vi "GetMeasurements (B fields first).vi"() -> ()   [LabVIEW 2016]
uses:
  <vilib>/Utility/file.llb/Write Delimited Spreadsheet (DBL).vi
panel:
  in  "DVM GIPB Address":string="7"
  out "# of Runs":i32=49
  in  "+B Field Removed?":bool
  out "Remove Field":bool
  out "# of Runs":i32=49
  in  "+B Field Added?":bool
  out "Ready To Change Field":bool
  out "# of Runs":i32
  in  "-B Field Added?":bool
  out "Ready To Change Field":bool
  in  "DVM resource name":refnum<visa-resource-name>="Keithley2128A"
  out "?":dbl=134.16905814972526
  out "Complete?":bool
  in  "Set Current (nA)":dbl=20.0 format="%.3f"
  in  "Voltage Measurement Path?":path=path "C:/Users/labuser/Desktop/KO Summer Research 19/Test/KO-Z2b.txt"
  in  "Current Source GPIB Address":string="12"
  # "SetUp DVM"
  # "minutes"
  # "3:"
  # "2:"
  # "1:"
  # "SetUp Current Source"
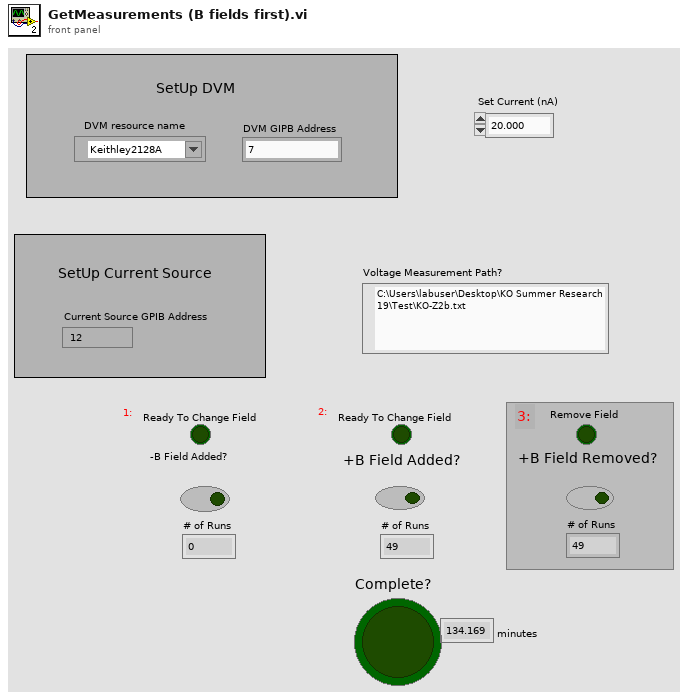
[diagram p1: front panel]
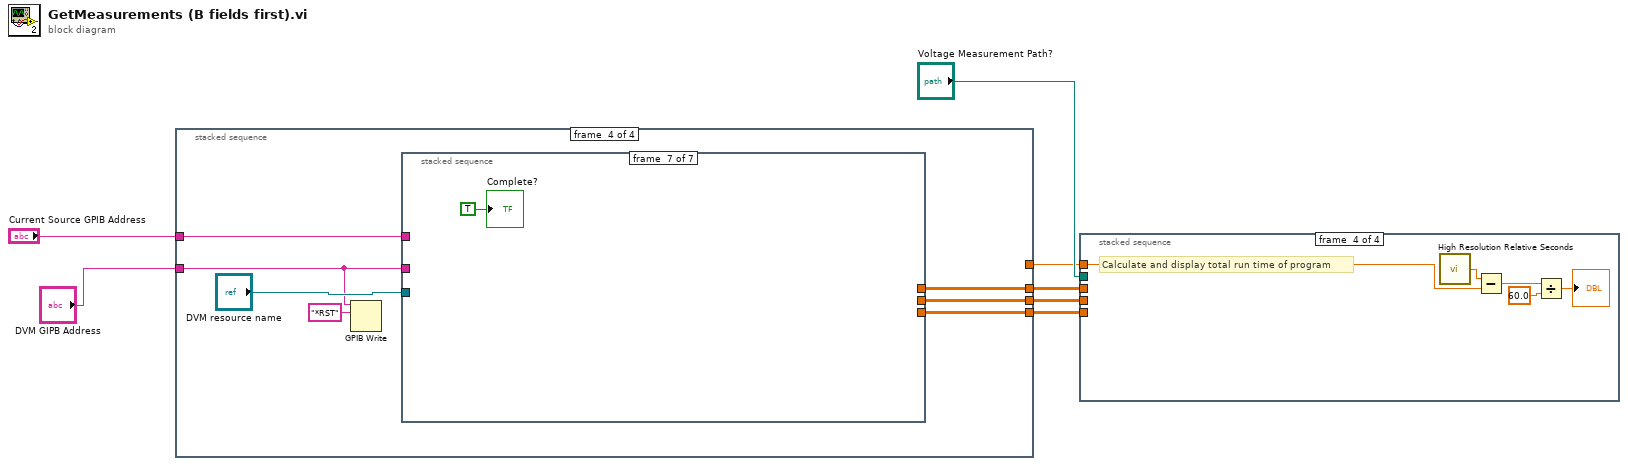
[diagram p0: block diagram]
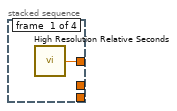
[diagram p2: hidden frame]
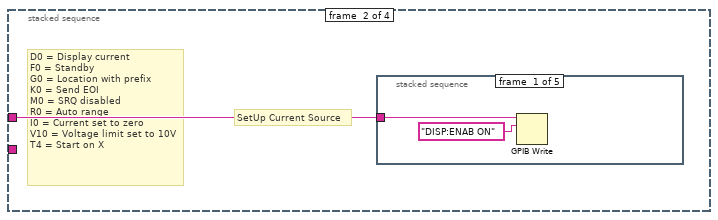
[diagram p3: hidden frame]
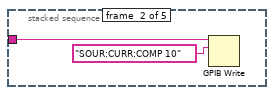
[diagram p4: hidden frame]
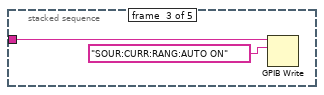
[diagram p5: hidden frame]
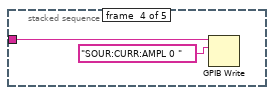
[diagram p6: hidden frame]
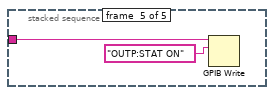
[diagram p7: hidden frame]
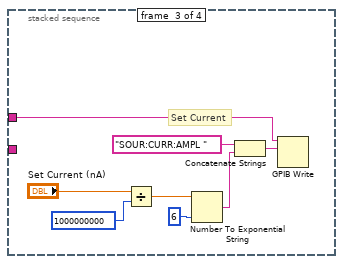
[diagram p8: hidden frame]
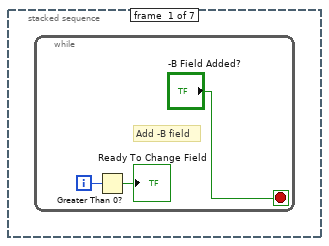
[diagram p9: hidden frame]
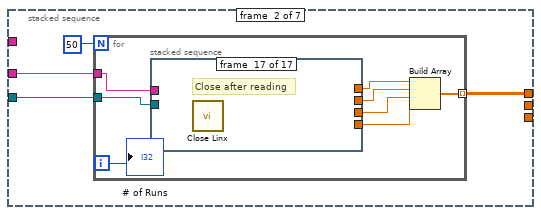
[diagram p10: hidden frame]
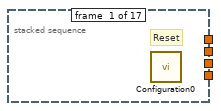
[diagram p11: hidden frame]
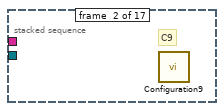
[diagram p12: hidden frame]
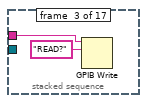
[diagram p13: hidden frame]
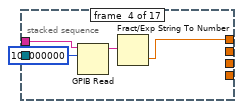
[diagram p14: hidden frame]
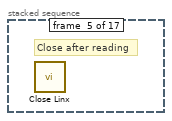
[diagram p15: hidden frame]
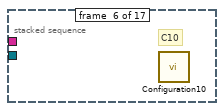
[diagram p16: hidden frame]
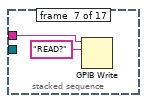
[diagram p17: hidden frame]
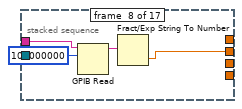
[diagram p18: hidden frame]
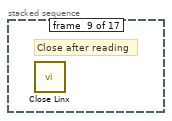
[diagram p19: hidden frame]
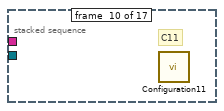
[diagram p20: hidden frame]
diagram:
  n1 = stacked-sequence {
    tunnel: "Current Source GPIB Address" -> [_ w9 w21 w34]
    tunnel: [w8 _ _ _] -> w5
    tunnel: [_ _ _ w33] -> w4
    tunnel: [_ _ _ w32] -> w3
    tunnel: [_ _ _ w31] -> w2
    tunnel: "DVM GIPB Address" -> [_ _ _ w28]
    frame #0 {
      n2 = call <vilib>:"High Resolution Relative Seconds.vi"() -> ("relative seconds"=w8:dbl)
    }
    frame #1 {
      # "SetUp Current Source"
      # "D0 = Display current\nF0 = Standby\nG0 = Location with prefix\nK0 = Send EOI\nM0 = SRQ disabled\nR0 = Auto range\nI0 = Current set to zero\nV10 = Voltage limit set to 10V\nT4 = Start on X"
      n3 = stacked-sequence {
        tunnel: w9 -> [w10 w12 w14 w16 w18]
        frame #0 {
          n4 = GPIB Write(0:w10, 1:"DISP:ENAB ON") -> ()  [unwired: 3 in, 2 out]
        }
        frame #1 {
          n5 = GPIB Write(0:w12, 1:"SOUR:CURR:COMP 10") -> ()  [unwired: 3 in, 2 out]
        }
        frame #2 {
          n6 = GPIB Write(0:w14, 1:"SOUR:CURR:RANG:AUTO ON") -> ()  [unwired: 3 in, 2 out]
        }
        frame #3 {
          n7 = GPIB Write(0:w16, 1:"SOUR:CURR:AMPL 0 ") -> ()  [unwired: 3 in, 2 out]
        }
        frame #4 {
          n8 = GPIB Write(0:w18, 1:"OUTP:STAT ON") -> ()  [unwired: 3 in, 2 out]
        }
      }
    }
    frame #2 {
      # "Set Current"
      n9 = Divide(x="Set Current (nA)", y=1000000000) -> (x/y=w23:dbl)
      n10 = Number To Exponential String(number=w23, precision (6)=6) -> (E-format string=w24:string)  [unwired: 2 in]
      n11 = Concatenate Strings("SOUR:CURR:AMPL ", w24) -> (w26:string)
      n12 = GPIB Write(0:w21, 1:w26) -> ()  [unwired: 3 in, 2 out]
    }
    frame #3 {
      n13 = GPIB Write(0:w28, 1:"*RST" ("data")) -> ()  [unwired: 3 in, 2 out]
      n14 = stacked-sequence {
        tunnel: w34 -> [_ _ _ _ _ w118 _]
        tunnel: [_ _ _ _ _ w117 _] -> w33
        tunnel: [_ w40 _ _ _ _ _] -> w32
        tunnel: [_ _ _ w80 _ _ _] -> w31
        tunnel: "DVM resource name" -> [_ w39 _ w78 _ w116 _]
        tunnel: w28 -> [_ w38 _ w77 _ w115 _]
        frame #0 {
          n15 = while {
            i -> [w36]
            stop <- "-B Field Added?" stop-if-true
            # "Add -B field"
            n16 = Greater Than 0?(x=w36) -> (x > 0?=→"Ready To Change Field":bool)
          }
        }
        frame #1 {
          n17 = for {
            N: 50 -> [_]
            tunnel: w39 -> [w48]
            tunnel: [w49] -> w40 mode=indexing
            tunnel: w38 -> [w42]
            i -> [w43]
            n18 = stacked-sequence {
              tunnel: w48 -> [_ _ _ _ _ _ _ _ _ _ _ _ _ _ _ _ _]
              tunnel: [_ _ _ w54 _ _ _ _ _ _ _ _ _ _ _ _ _] -> w47
              tunnel: [_ _ _ _ _ _ _ w59 _ _ _ _ _ _ _ _ _] -> w46
              tunnel: [_ _ _ _ _ _ _ _ _ _ _ w64 _ _ _ _ _] -> w45
              tunnel: [_ _ _ _ _ _ _ _ _ _ _ _ _ _ _ w70 _] -> w44
              tunnel: w42 -> [_ _ w51 w52 _ _ w57 w58 _ _ w63 w65 _ _ w69 w71 _]
              frame #0 {
                # "Reset"
                n19 = call "Configuration0.vi"() -> ()  [unwired: 12 in]
              }
              frame #1 {
                # "C9"
                n20 = call "Configuration9.vi"() -> ()  [unwired: 12 in]
              }
              frame #2 {
                n21 = GPIB Write(0:w51, 1:"READ?" ("data")) -> ()  [unwired: 3 in, 2 out]
              }
              frame #3 {
                n22 = GPIB Read(0:w52, 1:100000000 ("byte count")) -> (5:w55:string)  [unwired: 3 in, 2 out]
                n23 = Fract/Exp String To Number(string=w55) -> (number=w54:dbl)  [unwired: 3 in, 1 out]
              }
              frame #4 {
                # "Close after reading"
                n24 = call "Close Linx.vi"() -> ()  [unwired: 12 in]
              }
              frame #5 {
                # "C10"
                n25 = call "Configuration10.vi"() -> ()  [unwired: 12 in]
              }
              frame #6 {
                n26 = GPIB Write(0:w57, 1:"READ?" ("data")) -> ()  [unwired: 3 in, 2 out]
              }
              frame #7 {
                n27 = GPIB Read(0:w58, 1:100000000 ("byte count")) -> (5:w61:string)  [unwired: 3 in, 2 out]
                n28 = Fract/Exp String To Number(string=w61) -> (number=w59:dbl)  [unwired: 3 in, 1 out]
              }
              frame #8 {
                # "Close after reading"
                n29 = call "Close Linx.vi"() -> ()  [unwired: 12 in]
              }
              frame #9 {
                # "C11"
                n30 = call "Configuration11.vi"() -> ()  [unwired: 12 in]
              }
              frame #10 {
                n31 = GPIB Write(0:w63, 1:"READ?" ("data")) -> ()  [unwired: 3 in, 2 out]
              }
              frame #11 {
                n32 = GPIB Read(0:w65, 1:100000000 ("byte count")) -> (5:w67:string)  [unwired: 3 in, 2 out]
                n33 = Fract/Exp String To Number(string=w67) -> (number=w64:dbl)  [unwired: 3 in, 1 out]
              }
              frame #12 {
                # "Close after reading"
                n34 = call "Close Linx.vi"() -> ()  [unwired: 12 in]
              }
              frame #13 {
                # "C12"
                n35 = call "Configuration12.vi"() -> ()  [unwired: 12 in]
              }
              frame #14 {
                n36 = GPIB Write(0:w69, 1:"READ?" ("data")) -> ()  [unwired: 3 in, 2 out]
              }
              frame #15 {
                n37 = GPIB Read(0:w71, 1:100000000 ("byte count")) -> (5:w73:string)  [unwired: 3 in, 2 out]
                n38 = Fract/Exp String To Number(string=w73) -> (number=w70:dbl)  [unwired: 3 in, 1 out]
              }
              frame #16 {
                # "Close after reading"
                n39 = call "Close Linx.vi"() -> ()  [unwired: 12 in]
              }
            }
            n40 = Build Array(w47, w46, w45, w44) -> (w49:dbl[])
            "# of Runs" <- w43
          }
        }
        frame #2 {
          # "Change to +B Field"
          n41 = while {
            i -> [w74]
            stop <- "+B Field Added?" stop-if-true
            n42 = Greater Than 0?(x=w74) -> (x > 0?=→"Ready To Change Field":bool)
          }
        }
        frame #3 {
          n43 = for {
            N: 50 -> [_]
            tunnel: w78 -> [_]
            tunnel: [w87] -> w80 mode=indexing
            tunnel: w77 -> [w81]
            i -> [w86]
            n44 = stacked-sequence {
              tunnel: [_ _ _ w92 _ _ _ _ _ _ _ _ _ _ _ _ _] -> w85
              tunnel: [_ _ _ _ _ _ _ w97 _ _ _ _ _ _ _ _ _] -> w84
              tunnel: [_ _ _ _ _ _ _ _ _ _ _ _ _ _ _ w109 _] -> w82
              tunnel: [_ _ _ _ _ _ _ _ _ _ _ w103 _ _ _ _ _] -> w83
              tunnel: w81 -> [_ _ w88 w90 _ _ w94 w96 _ _ w100 w102 _ _ w106 w108 _]
              frame #0 {
                # "Reset"
                n45 = call "Configuration0.vi"() -> ()  [unwired: 12 in]
              }
              frame #1 {
                # "C13"
                n46 = call "Configuration9.vi"() -> ()  [unwired: 12 in]
              }
              frame #2 {
                n47 = GPIB Write(0:w88, 1:"READ?" ("data")) -> ()  [unwired: 3 in, 2 out]
              }
              frame #3 {
                n48 = GPIB Read(0:w90, 1:100000000 ("byte count")) -> (5:w93:string)  [unwired: 3 in, 2 out]
                n49 = Fract/Exp String To Number(string=w93) -> (number=w92:dbl)  [unwired: 3 in, 1 out]
              }
              frame #4 {
                # "Close after reading"
                n50 = call "Close Linx.vi"() -> ()  [unwired: 12 in]
              }
              frame #5 {
                # "C14"
                n51 = call "Configuration10.vi"() -> ()  [unwired: 12 in]
              }
              frame #6 {
                n52 = GPIB Write(0:w94, 1:"READ?" ("data")) -> ()  [unwired: 3 in, 2 out]
              }
              frame #7 {
                n53 = GPIB Read(0:w96, 1:100000000 ("byte count")) -> (5:w99:string)  [unwired: 3 in, 2 out]
                n54 = Fract/Exp String To Number(string=w99) -> (number=w97:dbl)  [unwired: 3 in, 1 out]
              }
              frame #8 {
                # "Close after reading"
                n55 = call "Close Linx.vi"() -> ()  [unwired: 12 in]
              }
              frame #9 {
                # "C15"
                n56 = call "Configuration11.vi"() -> ()  [unwired: 12 in]
              }
              frame #10 {
                n57 = GPIB Write(0:w100, 1:"READ?" ("data")) -> ()  [unwired: 3 in, 2 out]
              }
              frame #11 {
                n58 = GPIB Read(0:w102, 1:100000000 ("byte count")) -> (5:w105:string)  [unwired: 3 in, 2 out]
                n59 = Fract/Exp String To Number(string=w105) -> (number=w103:dbl)  [unwired: 3 in, 1 out]
              }
              frame #12 {
                # "Close after reading"
                n60 = call "Close Linx.vi"() -> ()  [unwired: 12 in]
              }
              frame #13 {
                # "C16"
                n61 = call "Configuration12.vi"() -> ()  [unwired: 12 in]
              }
              frame #14 {
                n62 = GPIB Write(0:w106, 1:"READ?" ("data")) -> ()  [unwired: 3 in, 2 out]
              }
              frame #15 {
                n63 = GPIB Read(0:w108, 1:100000000 ("byte count")) -> (5:w111:string)  [unwired: 3 in, 2 out]
                n64 = Fract/Exp String To Number(string=w111) -> (number=w109:dbl)  [unwired: 3 in, 1 out]
              }
              frame #16 {
                # "Close after reading"
                n65 = call "Close Linx.vi"() -> ()  [unwired: 12 in]
              }
            }
            n66 = Build Array(w85, w84, w83, w82) -> (w87:dbl[])
            "# of Runs" <- w86
          }
        }
        frame #4 {
          # "Change to +B Field"
          n67 = while {
            i -> [w112]
            stop <- "+B Field Removed?" stop-if-true
            n68 = Greater Than 0?(x=w112) -> (x > 0?=→"Remove Field":bool)
          }
        }
        frame #5 {
          # "Get Measurements"
          n69 = for {
            N: 50 -> [_]
            tunnel: [w130] -> w117 mode=indexing
            tunnel: w118 -> [_]
            tunnel: w116 -> [_]
            tunnel: w115 -> [w120]
            i -> [w129]
            # "Write"
            n70 = stacked-sequence {
              tunnel: [_ _ _ w135 _ _ _ _ _ _ _ _ _ _ _ _ _ _ _ _ _ _ _ _ _ _ _ _ _ _ _ _ _] -> w128
              tunnel: [_ _ _ _ _ _ _ w140 _ _ _ _ _ _ _ _ _ _ _ _ _ _ _ _ _ _ _ _ _ _ _ _ _] -> w127
              tunnel: [_ _ _ _ _ _ _ _ _ _ _ w146 _ _ _ _ _ _ _ _ _ _ _ _ _ _ _ _ _ _ _ _ _] -> w126
              tunnel: [_ _ _ _ _ _ _ _ _ _ _ _ _ _ _ w152 _ _ _ _ _ _ _ _ _ _ _ _ _ _ _ _ _] -> w125
              tunnel: [_ _ _ _ _ _ _ _ _ _ _ _ _ _ _ _ _ _ _ w158 _ _ _ _ _ _ _ _ _ _ _ _ _] -> w124
              tunnel: [_ _ _ _ _ _ _ _ _ _ _ _ _ _ _ _ _ _ _ _ _ _ _ w164 _ _ _ _ _ _ _ _ _] -> w123
              tunnel: [_ _ _ _ _ _ _ _ _ _ _ _ _ _ _ _ _ _ _ _ _ _ _ _ _ _ _ w170 _ _ _ _ _] -> w122
              tunnel: [_ _ _ _ _ _ _ _ _ _ _ _ _ _ _ _ _ _ _ _ _ _ _ _ _ _ _ _ _ _ _ w176 _] -> w121
              tunnel: w120 -> [_ _ w131 w133 _ _ w137 w139 _ _ w143 w145 _ _ w149 w151 _ _ w155 w157 _ _ w161 w163 _ _ w167 w169 _ _ w173 w175 _]
              frame #0 {
                # "Reset"
                n71 = call "Configuration0.vi"() -> ()  [unwired: 12 in]
              }
              frame #1 {
                # "C1"
                n72 = call "Configuration1.vi"() -> ()  [unwired: 12 in]
              }
              frame #2 {
                n73 = GPIB Write(0:w131, 1:"READ?" ("data")) -> ()  [unwired: 3 in, 2 out]
              }
              frame #3 {
                n74 = GPIB Read(0:w133, 1:100000000 ("byte count")) -> (5:w136:string)  [unwired: 3 in, 2 out]
                n75 = Fract/Exp String To Number(string=w136) -> (number=w135:dbl)  [unwired: 3 in, 1 out]
              }
              frame #4 {
                # "Close after reading"
                n76 = call "Close Linx.vi"() -> ()  [unwired: 12 in]
              }
              frame #5 {
                # "C2"
                n77 = call "Configuration2.vi"() -> ()  [unwired: 12 in]
              }
              frame #6 {
                n78 = GPIB Write(0:w137, 1:"READ?" ("data")) -> ()  [unwired: 3 in, 2 out]
              }
              frame #7 {
                n79 = GPIB Read(0:w139, 1:100000000 ("byte count")) -> (5:w142:string)  [unwired: 3 in, 2 out]
                n80 = Fract/Exp String To Number(string=w142) -> (number=w140:dbl)  [unwired: 3 in, 1 out]
              }
              frame #8 {
                # "Close after reading"
                n81 = call "Close Linx.vi"() -> ()  [unwired: 12 in]
              }
              frame #9 {
                # "C3"
                n82 = call "Configuration3.vi"() -> ()  [unwired: 12 in]
              }
              frame #10 {
                n83 = GPIB Write(0:w143, 1:"READ?" ("data")) -> ()  [unwired: 3 in, 2 out]
              }
              frame #11 {
                n84 = GPIB Read(0:w145, 1:100000000 ("byte count")) -> (5:w148:string)  [unwired: 3 in, 2 out]
                n85 = Fract/Exp String To Number(string=w148) -> (number=w146:dbl)  [unwired: 3 in, 1 out]
              }
              frame #12 {
                # "Close after reading"
                n86 = call "Close Linx.vi"() -> ()  [unwired: 12 in]
              }
              frame #13 {
                # "C4"
                n87 = call "Configuration4.vi"() -> ()  [unwired: 12 in]
              }
              frame #14 {
                n88 = GPIB Write(0:w149, 1:"READ?" ("data")) -> ()  [unwired: 3 in, 2 out]
              }
              frame #15 {
                n89 = GPIB Read(0:w151, 1:100000000 ("byte count")) -> (5:w154:string)  [unwired: 3 in, 2 out]
                n90 = Fract/Exp String To Number(string=w154) -> (number=w152:dbl)  [unwired: 3 in, 1 out]
              }
              frame #16 {
                # "Close after reading"
                n91 = call "Close Linx.vi"() -> ()  [unwired: 12 in]
              }
              frame #17 {
                # "C5"
                n92 = call "Configuration5.vi"() -> ()  [unwired: 12 in]
              }
              frame #18 {
                n93 = GPIB Write(0:w155, 1:"READ?" ("data")) -> ()  [unwired: 3 in, 2 out]
              }
              frame #19 {
                n94 = GPIB Read(0:w157, 1:100000000 ("byte count")) -> (5:w160:string)  [unwired: 3 in, 2 out]
                n95 = Fract/Exp String To Number(string=w160) -> (number=w158:dbl)  [unwired: 3 in, 1 out]
              }
              frame #20 {
                # "Close after reading"
                n96 = call "Close Linx.vi"() -> ()  [unwired: 12 in]
              }
              frame #21 {
                # "C6"
                n97 = call "Configuration6.vi"() -> ()  [unwired: 12 in]
              }
              frame #22 {
                n98 = GPIB Write(0:w161, 1:"READ?" ("data")) -> ()  [unwired: 3 in, 2 out]
              }
              frame #23 {
                n99 = GPIB Read(0:w163, 1:100000000 ("byte count")) -> (5:w166:string)  [unwired: 3 in, 2 out]
                n100 = Fract/Exp String To Number(string=w166) -> (number=w164:dbl)  [unwired: 3 in, 1 out]
              }
              frame #24 {
                # "Close after reading"
                n101 = call "Close Linx.vi"() -> ()  [unwired: 12 in]
              }
              frame #25 {
                # "C7"
                n102 = call "Configuration7.vi"() -> ()  [unwired: 12 in]
              }
              frame #26 {
                n103 = GPIB Write(0:w167, 1:"READ?" ("data")) -> ()  [unwired: 3 in, 2 out]
              }
              frame #27 {
                n104 = GPIB Read(0:w169, 1:100000000 ("byte count")) -> (5:w172:string)  [unwired: 3 in, 2 out]
                n105 = Fract/Exp String To Number(string=w172) -> (number=w170:dbl)  [unwired: 3 in, 1 out]
              }
              frame #28 {
                # "Close after reading"
                n106 = call "Close Linx.vi"() -> ()  [unwired: 12 in]
              }
              frame #29 {
                # "C8"
                n107 = call "Configuration8.vi"() -> ()  [unwired: 12 in]
              }
              frame #30 {
                n108 = GPIB Write(0:w173, 1:"READ?" ("data")) -> ()  [unwired: 3 in, 2 out]
              }
              frame #31 {
                n109 = GPIB Read(0:w175, 1:100000000 ("byte count")) -> (5:w178:string)  [unwired: 3 in, 2 out]
                n110 = Fract/Exp String To Number(string=w178) -> (number=w176:dbl)  [unwired: 3 in, 1 out]
              }
              frame #32 {
                # "Close after reading"
                n111 = call "Close Linx.vi"() -> ()  [unwired: 12 in]
              }
            }
            n112 = Build Array(w128, w127, w126, w125, w124, w123, w122, w121) -> (w130:dbl[])
            "# of Runs" <- w129
          }
        }
        frame #6 {
          "Complete?" <- TRUE
        }
      }
    }
  }
  n113 = stacked-sequence {
    tunnel: "Voltage Measurement Path?" -> [w181 w187 w193 _]
    tunnel: w4 -> [w180 _ _ _]
    tunnel: w3 -> [_ w186 _ _]
    tunnel: w5 -> [_ _ _ w198]
    tunnel: w2 -> [_ _ w192 _]
    frame #0 {
      # "Write voltages (V) to file (.txt)"
      n114 = call-poly <vilib>:"Write Delimited Spreadsheet.vi"("file path (dialog if empty)"=w181, "format (%.3f)"="%16.14f", "2D data"=w180, "append to file? (new file:F)"=TRUE ("append to file? (F)"), "transpose? (no:F)"=FALSE ("transpose? (F)"), "delimiter (\\t)"="," ("delimiter (\\t)")) -> ()  [unwired: 8 in, 2 out]
    }
    frame #1 {
      # "Write voltages (V) to file (.txt)"
      n115 = call-poly <vilib>:"Write Delimited Spreadsheet.vi"("file path (dialog if empty)"=w187, "format (%.3f)"="%16.14f", "2D data"=w186, "append to file? (new file:F)"=TRUE ("append to file? (F)"), "transpose? (no:F)"=FALSE ("transpose? (F)"), "delimiter (\\t)"="," ("delimiter (\\t)")) -> ()  [unwired: 8 in, 2 out]
    }
    frame #2 {
      n116 = call-poly <vilib>:"Write Delimited Spreadsheet.vi"("file path (dialog if empty)"=w193, "format (%.3f)"="%16.14f", "2D data"=w192, "append to file? (new file:F)"=TRUE ("append to file? (F)"), "transpose? (no:F)"=FALSE ("transpose? (F)"), "delimiter (\\t)"="," ("delimiter (\\t)")) -> ()  [unwired: 8 in, 2 out]
    }
    frame #3 {
      # "Calculate and display total run time of program"
      n117 = call <vilib>:"High Resolution Relative Seconds.vi"() -> ("relative seconds"=w202:dbl)
      n118 = Subtract(x=w202, y=w198) -> (x-y=w201:dbl)
      n119 = Divide(x=w201, y=60.0) -> (x/y=→"?":dbl)
    }
  }
